vi "test_MultipleSessionsReserved_CallCloseSessionsTwice_CloseNotCalledSecondTime.vi"(8 "error in":errorcluster) -> (0 "error out":errorcluster, 2 "result":string, 3 "pass":bool)   [LabVIEW 2020, in "MeasurementServerTests.lvlib"]
uses:
  MeasurementServerTests.lvlib
  Helpers/Fake Session Factory/Call Recorder Action.ctl
  Runtime/Clients/Session Management V1/Session Reservation/Session Reservation.lvclass
  Helpers/Fake Session Factory/Fake Session Factory.lvclass
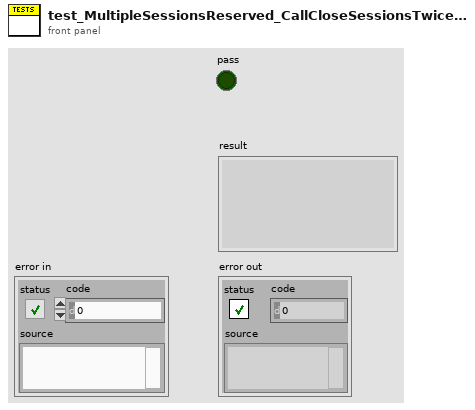
[diagram p1: front panel]
types:
  T1 = typedef "MeasurementServerTests.lvlib/Fake Session Factory.lvclass/Call Recorder Action.ctl" = enum16{"Initialize", "Read Values", "Record Initialize-Initialize", "Record Initialize-Attach", "Record Close-Close", "Record Close-Detach"}
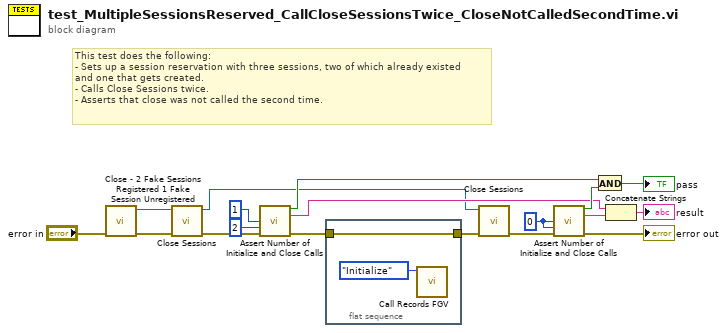
[diagram p0: block diagram]
diagram:
  w10 = u32 0 ("expected close-close calls")
  # "This test does the following:\n- Sets up a session reservation with three sessions, two of which already existed\nand one that gets created.\n- Calls Close Sessions twice.\n- Asserts that close was not called the second time."
  n1 = call "Close - 2 Fake Sessions Registered 1 Fake Session Unregistered.vi"("error in"="error in") -> ("error out"=w17:errorcluster, "session reservation out"=w16:refnum<class "Session Reservation.lvclass">)  [unwired: 9 in]
  n2 = call "Close Sessions.vi"("error in"=w17, "session reservation in"=w16) -> ("error out"=w15:errorcluster, "session reservation out"=w3:refnum<class "Session Reservation.lvclass">)  [unwired: 8 in]
  n3 = call "Assert Number of Initialize and Close Calls.vi"("expected close-close calls"=u32 1, "expected close-detach calls"=u32 2, "error in"=w15) -> ("pass"=w7:bool, "result"=w5:string, "error out"=w2:errorcluster)  [unwired: 10 in]
  n4 = flat-sequence {
    tunnel: w2 -> [w20]
    tunnel: [w20] -> w1
    frame #0 {
      n5 = call "Call Records FGV.vi"("call recorder action"=Call_Recorder_Action."Initialize" ("Call Recorder Action")) -> ()  [unwired: 7 in, 4 out]
    }
  }
  n6 = call "Close Sessions.vi"("error in"=w1, "session reservation in"=w3) -> ("error out"=w12:errorcluster)  [unwired: 8 in, 1 out]
  n7 = call "Assert Number of Initialize and Close Calls.vi"("expected close-close calls"=w10, "expected close-detach calls"=w10, "error in"=w12) -> ("pass"=w9:bool, "result"=w6:string, "error out"=→"error out":errorcluster)  [unwired: 10 in]
  n8 = And(x=w7, y=w9) -> (x .and. y?=→"pass":bool)
  n9 = Concatenate Strings(w5, w6) -> (→"result":string)
